vi "Write Name.vi"(10 "Name":string, 11 "(WavIndex_Pointer) in":refnum<class "(WavIndex_Pointer).lvclass">) -> (3 "(WavIndex_Pointer) out":refnum<class "(WavIndex_Pointer).lvclass">)   [LabVIEW 2016, in "(WavIndex_Pointer).lvclass"]
uses:
  (WavIndex_Pointer).lvclass
  (WavIndex_Pointer).lvclass/(WavIndex_Pointer).ctl
  ((Pointer)).lvclass
  Index_Pointer/(Index_Pointer).lvclass
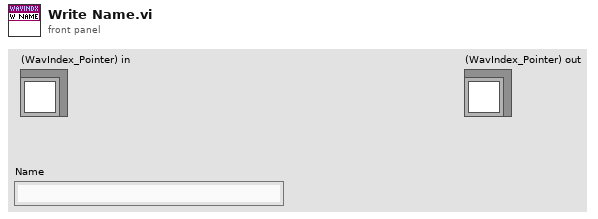
[diagram p1: front panel]
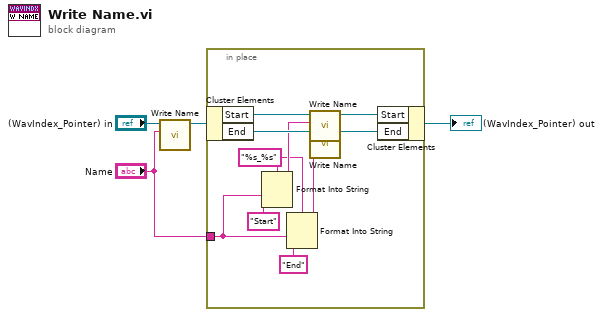
[diagram p0: block diagram]
diagram:
  n1 = call-parent "Write Name.vi"("Name"="Name", "((Pointer)) in"="(WavIndex_Pointer) in") -> ("((Pointer)) out"=w3:refnum<class "(WavIndex_Pointer).lvclass">)  [unwired: 9 in]
  n2 = in-place {
    in-place-border: "Name" -> [w5]
    w9 = "%s_%s" ("format string")
    n3 = in-place-cluster #1(w3) -> ("Start"=w13:refnum<class "(Index_Pointer).lvclass">, "End"=w14:refnum<class "(Index_Pointer).lvclass">)
    n4 = Format Into String(format string=w9, w5, "Start") -> (resulting string=w10:string)  [unwired: 2 in, 1 out]
    n5 = Format Into String(format string=w9, w5, "End") -> (resulting string=w8:string)  [unwired: 2 in, 1 out]
    n6 = call-dynamic "Write Name.vi"("Name"=w10, "(Index_Pointer) in"=w13) -> ("(Index_Pointer) out"=w12:refnum<class "(Index_Pointer).lvclass">)  [unwired: 9 in]
    n7 = call-dynamic "Write Name.vi"("Name"=w8, "(Index_Pointer) in"=w14) -> ("(Index_Pointer) out"=w11:refnum<class "(Index_Pointer).lvclass">)  [unwired: 9 in]
    n8 = in-place-cluster #1("Start"=w12, "End"=w11) -> (→"(WavIndex_Pointer) out":refnum<class "(WavIndex_Pointer).lvclass">)
  }
